vi "GetMainGUIFlags.vi"(8 "error in (no error)":errorcluster, 11 "TestSeqClass in":refnum<class "TestSeqClass.lvclass">) -> (0 "error out":errorcluster, 1 "Flags":cluster{"Exit":bool}, 3 "TestSeqClass out":refnum<class "TestSeqClass.lvclass">)   [LabVIEW 2019, in "TestSeqClass.lvclass"]
uses:
  TestSeqClass.lvclass
  GUIHandler_Main/GUI_Handler_Main.lvclass/GUI_Handler_Main.ctl
  GUIHandler_Main/GUI_Handler_Main.lvclass
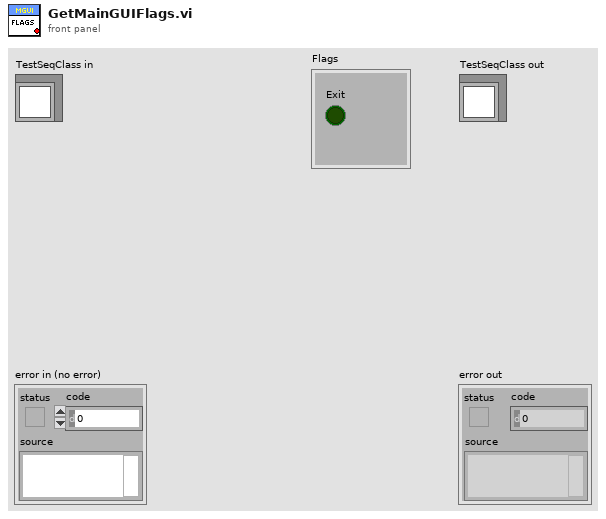
[diagram p1: front panel]
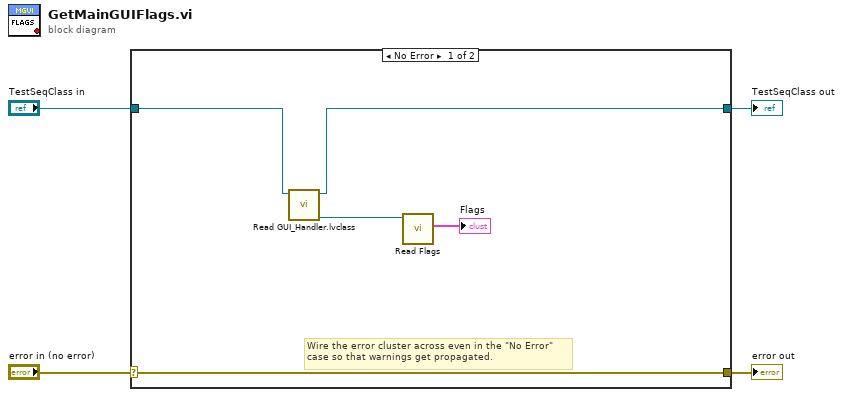
[diagram p0: block diagram]
diagram:
  n1 = case shown="No Error" "error in (no error)" {
    selector: "error in (no error)" -> [w9 w11]
    tunnel: [w9 w11] -> w3
    tunnel: [w6 w10] -> w1
    tunnel: "TestSeqClass in" -> [w7 w10]
    frame No Error {
      # "Wire the error cluster across even in the \"No Error\"\ncase so that warnings get propagated."
      n2 = call-dynamic "Read GUI_Handler.lvclass.vi"("TestSeqClass in"=w7) -> ("GUI_Handler.lvclass"=w8:refnum<class "GUI_Handler_Main.lvclass">, "TestSeqClass out"=w6:refnum<class "TestSeqClass.lvclass">)  [unwired: 8 in, 1 out]
      n3 = call "Read Flags.vi"("GUI_Handler_Main in"=w8) -> ("Flags"=→"Flags":cluster{"Exit":bool})  [unwired: 8 in, 2 out]
    }
    frame Error {
    }
  }
  "error out" <- w3
  "TestSeqClass out" <- w1
